vi "Method.vi"(4 "Input B":refnum<class "Abs_Numeric.lvclass">, 5 "Input A":T1) -> (1 "Result":T1)   [LabVIEW 2021, in "Multiply_CPLX_SGL.lvclass"]
uses:
  Multiply_CPLX_SGL.lvclass
  Abs_Type.ctl
  Abs_Types/Complex Single Float/Complex Single Float.lvclass
  Abs_Types/Numeric/Abs_Numeric.lvclass
  C:/Users/Tim/Documents/LabVIEW/2021/Data Classes/Source/Functions/Support/Two Terminal/Cmplx SGL/AbsFunc_Two Term_Complex SGL.lvclass
  C:/Users/Tim/Documents/LabVIEW/2021/Data Classes/Source/Abs_Types/Complex Single Float/Complex Single Float.lvclass
  Support/Two Terminal/Cmplx SGL/AbsFunc_Two Term_Complex SGL.lvclass/AbsFunc_Two Term_Complex SGL.ctl
  Support/Two Terminal/Cmplx SGL/Properties/Write Numeric A.vi
  Support/Two Terminal/Cmplx SGL/Properties/Write Numeric B.vi
  Multiply_CPLX_SGL.lvclass/Multiply_CPLX_SGL.ctl
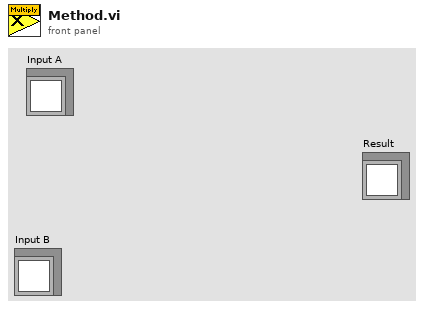
[diagram p1: front panel]
types:
  T1 = typedef "Multiply_CPLX_SGL.lvclass/Abs_Type.ctl" = refnum<class "Complex Single Float.lvclass">
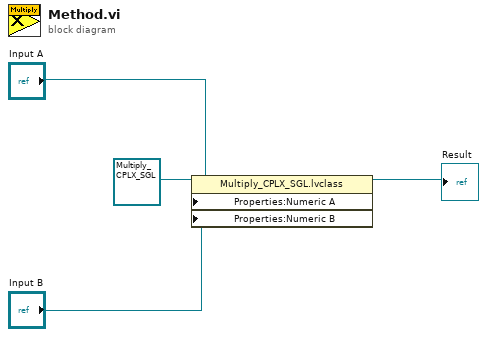
[diagram p0: block diagram]
diagram:
  n1 = property class="Multiply_CPLX_SGL.lvclass"(reference=refnum<class "Multiply_CPLX_SGL.lvclass"> refnum ("Functions.lvlib:Numeric.lvlib:Multiply.lvclass"), "Properties:Numeric A"="Input A", "Properties:Numeric B"="Input B") -> (reference out=→"Result":refnum<class "Multiply_CPLX_SGL.lvclass">)  [unwired: 1 in, 1 out]
